vi "Construct Connection Factory Session.vi"(10 "Log Instance":refnum<class "LoggerReference.lvclass">, 11 "Connection Factory Type":refnum<class "IConnectionFactory.lvclass">) -> (0 "error out":errorcluster, 3 "Connection Factory Session":refnum<data-value>)   [LabVIEW 2019, in "ConnectionFactorySession.lvlib" / "ConnectionFactorySession.lvclass"]
uses:
  <vilib>/gpm_packages/@cs/Network-interface/Source/Connection Factory Session/ConnectionFactorySession/ConnectionFactorySession.lvclass
  <vilib>/gpm_packages/@cs/Network-interface/Source/IConnectionFactory/IConnectionFactory.lvclass
  <vilib>/gpm_packages/@cs/event-logger/Source/Composed Log/LoggerReference/LoggerReference.lvclass
  <vilib>/gpm_packages/@cs/Network-interface/Source/Connection Factory Session/ConnectionFactoryHandler/ConnectionFactoryHandler.lvclass/ConnectionFactoryHandler.ctl
  <vilib>/gpm_packages/@cs/Network-interface/Source/Logged Actor/LoggedActor.lvclass/LoggedActor.ctl
  <vilib>/gpm_packages/@cs/Network-interface/Source/Connection Factory Session/ConnectionFactorySession/ConnectionFactorySession.lvclass/ConnectionFactorySession.ctl
  <vilib>/gpm_packages/@cs/Network-interface/Source/Create Ref Message/Create Ref Message.lvclass/Create Ref Message.ctl
  <vilib>/ActorFramework/Message Enqueuer/Message Enqueuer.lvclass/Message Enqueuer.ctl
  <vilib>/gpm_packages/@cs/Network-interface/Source/Logged Actor/Set Log Instance and ID.vi
  <vilib>/ActorFramework/Message Enqueuer/Enqueue.vi
  <vilib>/gpm_packages/@cs/Network-interface/Source/Connection Factory Session/ConnectionFactoryHandler/ConnectionFactoryHandler.lvclass
  C:/Program Files/National Instruments/LabVIEW 2019/vi.lib/gpm_packages/@cs/Network-interface/Source/Logged Actor/LoggedActor.lvclass
  C:/Program Files/National Instruments/LabVIEW 2019/vi.lib/ActorFramework/Actor/Actor.lvclass
  <vilib>/gpm_packages/@cs/Network-interface/Source/Create Ref Message/Create Ref Message.lvclass
  C:/Program Files/National Instruments/LabVIEW 2019/vi.lib/ActorFramework/Message/Message.lvclass
  <vilib>/ActorFramework/Message Priority Queue/Priority Enqueue.vi
  <vilib>/ActorFramework/Actor/Actor.lvclass
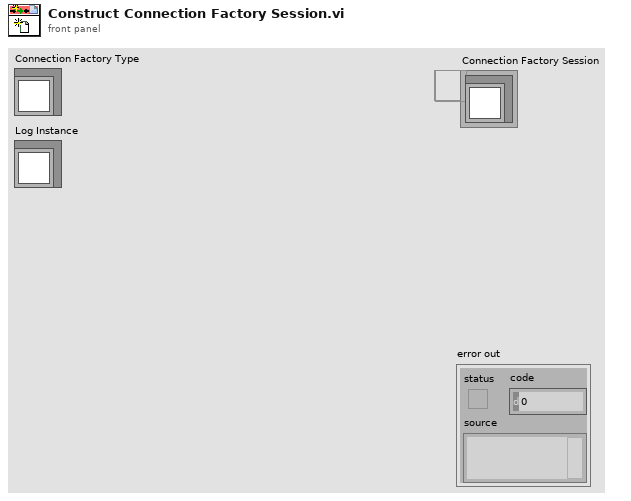
[diagram p1: front panel]
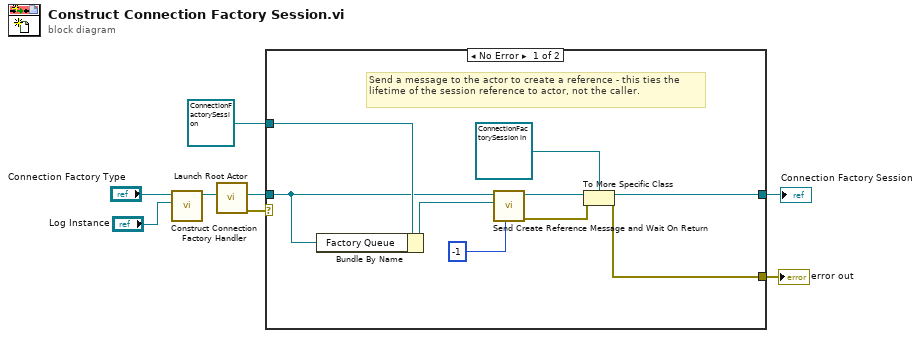
[diagram p0: block diagram]
diagram:
  n1 = call <vilib>:"Construct Connection Factory Handler.vi"("Log Instance"="Log Instance", "Connection Factory Type"="Connection Factory Type") -> ("ConnectionFactoryHandler"=w7:refnum<class "ConnectionFactoryHandler.lvclass">)  [unwired: 9 in]
  n2 = call <vilib>:"Launch Root Actor.vi"("Actor"=w7) -> ("error out"=w5:errorcluster, "Actor's Enqueuer"=w6:refnum<class "Message Enqueuer.lvclass">)  [unwired: 9 in]
  n3 = case shown="No Error" w5 {
    selector: w5 -> [_ w18]
    tunnel: refnum<class "ConnectionFactorySession.lvclass"> refnum ("ConnectionFactorySession in") -> [w17 _]
    tunnel: w6 -> [w16 _]
    tunnel: [w10 w18] -> w3
    tunnel: [w9 _] -> w2
    frame No Error {
      # "Send a message to the actor to create a reference - this ties the lifetime of the session reference to actor, not the caller."
      n4 = Bundle By Name(cluster=w17, "Factory Queue"=w16) -> (w15:refnum<class "ConnectionFactorySession.lvclass">)
      n5 = call <vilib>:"Send Create Reference Message and Wait On Return.vi"("timeout in ms (-1)"=-1, "Object"=w15, "Message Enqueuer in"=w16) -> ("error out"=w11:errorcluster, "Object Reference"=w13:refnum<data-value>)  [unwired: 7 in]
      n6 = To More Specific Class(target class=refnum<data-value> refnum ("data value reference"), reference=w13, error in=w11) -> (specific class reference=w9:refnum<data-value>, error out=w10:errorcluster)
    }
    frame Error {
    }
  }
  "error out" <- w3
  "Connection Factory Session" <- w2
